vi "B.vi"(3 "t":dbl, 4 "n^2":dbl, 5 "Promien krzywizny południka":dbl, 6 "fi[rad]":dbl) -> (0 "B":dbl)   [LabVIEW 2015, in "Biblioteka moduł map v3.lvlib" / "Konwersja wsp.lvlib" / "UTM.lvlib" / "Konwersja na UTM.lvlib"]
doc: "Współczynnik wzoru na konwersję na UTM."
uses:
  Konwersja na UTM.lvlib
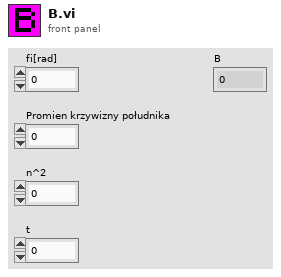
[diagram p1: front panel]
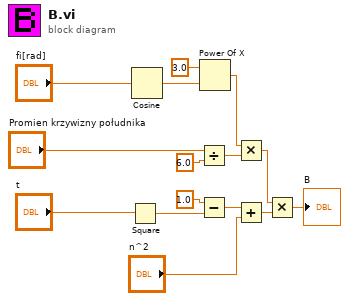
[diagram p0: block diagram]
diagram:
  n1 = Square(x="t") -> (x^2=w9:dbl)
  n2 = Cosine(x="fi[rad]") -> (cos(x)=w4:dbl)
  n3 = Divide(x="Promien krzywizny południka", y=6.0) -> (x/y=w7:dbl)
  n4 = Subtract(x=1.0, y=w9) -> (x-y=w11:dbl)
  n5 = Power Of X(1:w4, 2:3.0 ("y")) -> (0:w6:dbl)
  n6 = Multiply(x=w6, y=w7) -> (x*y=w13:dbl)
  n7 = Add(x=w11, y="n^2") -> (x+y=w14:dbl)
  n8 = Multiply(x=w13, y=w14) -> (x*y=→"B":dbl)
